vi "addProperty.vi"(8 "error in (no error)":errorcluster, 10 "Property in":refnum<class "IProperty.lvclass">, 11 "IPropertyObject in":refnum<class "IPropertyObject.lvclass">) -> (0 "error out":errorcluster, 2 "Property out":refnum<class "IProperty.lvclass">, 3 "IPropertyObject out":refnum<class "IPropertyObject.lvclass">)   [LabVIEW 2022 SP3, in "openDAQ.lvlib" / "IBaseObject.lvlib" / "IPropertyObject.lvlib" / "IPropertyObject.lvclass"]
uses:
  <instrlib>/openDAQ/Public/Classes/IPropertyObject/IPropertyObject.lvclass
  <instrlib>/openDAQ/Public/Classes/IPropertyObject/IPropertyObject.lvclass/IPropertyObject.ctl
  <instrlib>/openDAQ/Public/Classes/IProperty/IProperty.lvclass
  <instrlib>/openDAQ/Binaries/Windows/x86/copendaq32.dll
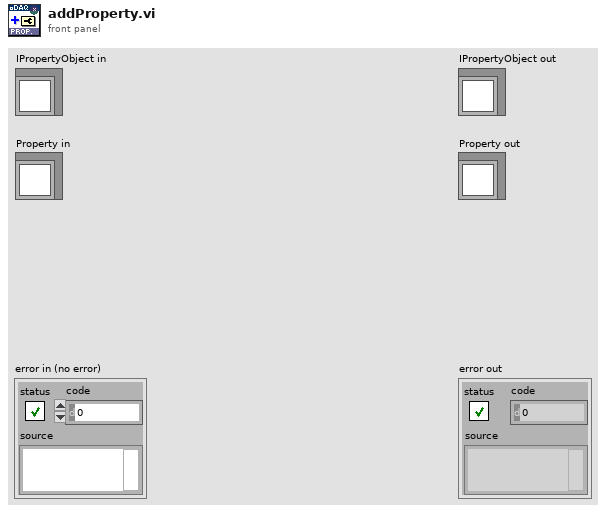
[diagram p1: front panel]
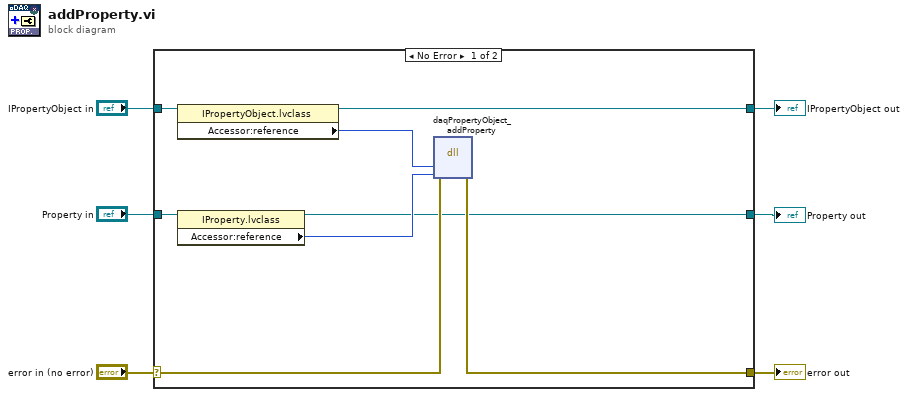
[diagram p0: block diagram]
diagram:
  n1 = case shown="No Error" "error in (no error)" {
    selector: "error in (no error)" -> [w14 w17]
    tunnel: [w13 w17] -> w5
    tunnel: [w10 w16] -> w3
    tunnel: "IPropertyObject in" -> [w12 w16]
    tunnel: "Property in" -> [w9 w15]
    tunnel: [w7 w15] -> w1
    frame No Error {
      n2 = property class="IPropertyObject.lvclass"(reference=w12) -> (reference out=w10:refnum<class "IPropertyObject.lvclass">, "Accessor:reference"=w11:i64)  [unwired: 1 in, 1 out]
      n3 = property class="IProperty.lvclass"(reference=w9) -> (reference out=w7:refnum<class "IProperty.lvclass">, "Accessor:reference"=w8:i64)  [unwired: 1 in, 1 out]
      n4 = dll-call lib="C:/Program Files (x86)/National Instruments/LabVIEW 2022/instr.lib/openDAQ/Binaries/Windows/x86/copendaq*.*" fn="daqPropertyObject_addProperty"(error in=w14, "PropertyObject"=w11, "Property"=w8) -> (error out=w13:errorcluster)  [unwired: 5 in, 1 out]
    }
    frame Error {
    }
  }
  "error out" <- w5
  "IPropertyObject out" <- w3
  "Property out" <- w1
